vi "SetConf.vi"(8 "error in (no error)":errorcluster, 11 "BME68x in":refnum<class "BME680.lvclass">) -> (0 "error out":errorcluster, 3 "BME68x out":refnum<class "BME680.lvclass">)   [LabVIEW 2022 SP3, in "BME680.lvlib" / "BME680.lvclass"]
uses:
  BME680.lvclass
  BME680.lvclass/BME680.ctl
  Typedefs/Conf.ctl
panel:
  in  "Conf":T1
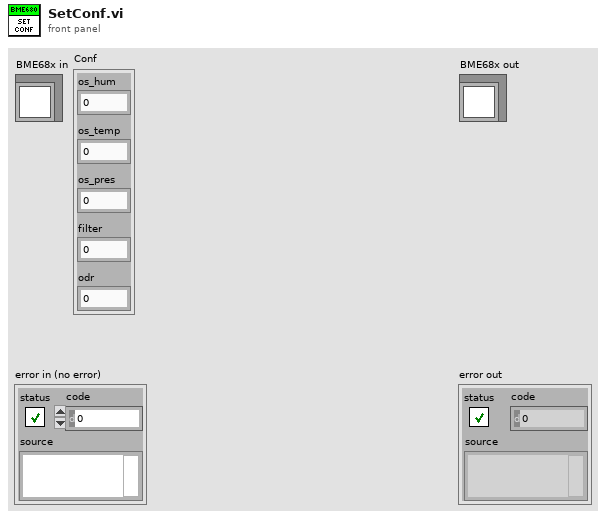
[diagram p1: front panel]
types:
  T1 = typedef "BME680.lvlib/BME680.lvclass/Conf.ctl" = cluster{"os_hum":u8, "os_temp":u8, "os_pres":u8, "filter":u8, "odr":u8}
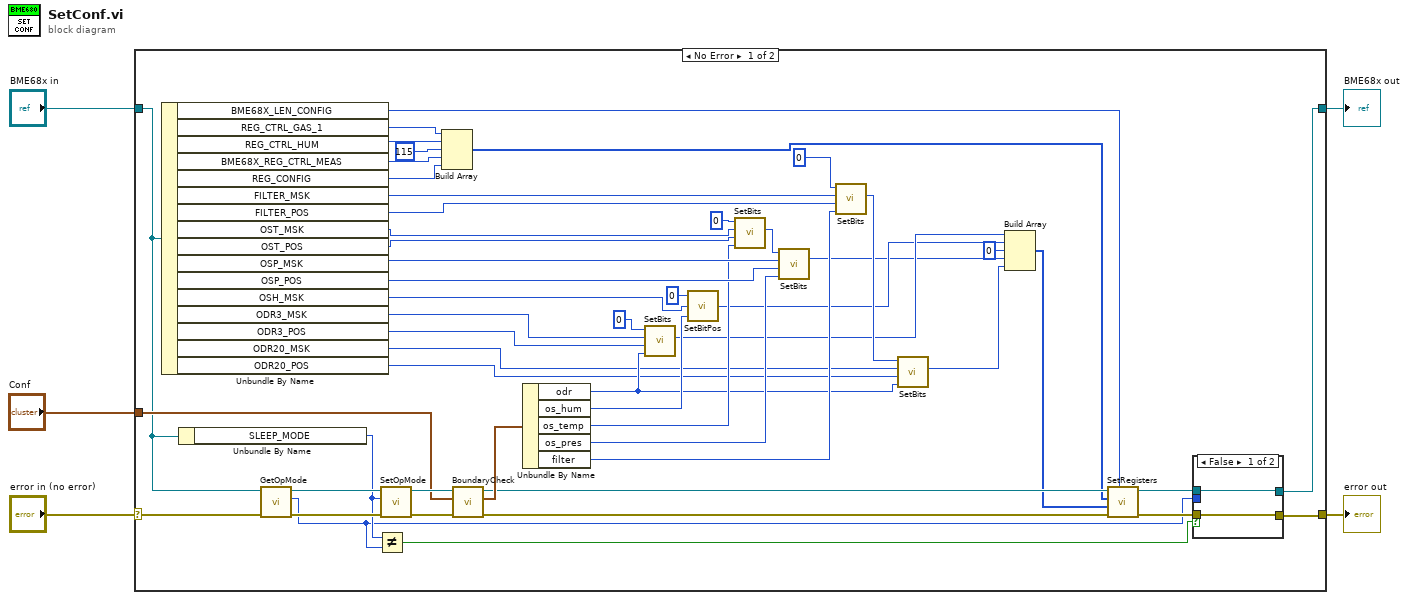
[diagram p0: block diagram]
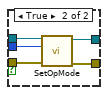
[diagram p2: hidden frame]
diagram:
  n1 = case shown="No Error" "error in (no error)" {
    selector: "error in (no error)" -> [w57 w66]
    tunnel: [w7 w66] -> w4
    tunnel: [w6 w65] -> w2
    tunnel: "BME68x in" -> [w51 w65]
    tunnel: "Conf" -> [w52 _]
    frame No Error {
      n2 = Unbundle By Name(w51) -> ("BME68X_LEN_CONFIG"=w15:u8, "REG_CTRL_GAS_1"=w50:u8, "REG_CTRL_HUM"=w49:u8, "BME68X_REG_CTRL_MEAS"=w48:u8, "REG_CONFIG"=w47:u8, "FILTER_MSK"=w42:u8, "FILTER_POS"=w41:u8, "OST_MSK"=w40:u8, "OST_POS"=w39:u8, "OSP_MSK"=w37:u8, "OSP_POS"=w36:u8, "OSH_MSK"=w34:u8, "ODR3_MSK"=w28:u8, "ODR3_POS"=w27:u8, "ODR20_MSK"=w26:u8, "ODR20_POS"=w25:u8)
      n3 = Unbundle By Name(w51) -> ("SLEEP_MODE"=w10:u8)
      n4 = call-dynamic "GetOpMode.vi"("error in (no error)"=w57, "BME680 in"=w51) -> ("error out"=w56:errorcluster, "Op Mode"=w9:u8, "BME680 out"=w55:refnum<class "BME680.lvclass">)  [unwired: 7 in]
      n5 = Not Equal?(x=w10, y=w9) -> (x != y?=w8:bool)
      n6 = call-dynamic "SetOpMode.vi"("error in (no error)"=w56, "Op Mode"=w10, "BME680 in"=w55) -> ("error out"=w54:errorcluster, "BME680 out"=w53:refnum<class "BME680.lvclass">)  [unwired: 7 in]
      n7 = Build Array(w50, w49, u8 115 ("element"), w48, w47) -> (w14:u8[])
      n8 = call "BoundaryCheck.vi"("error in (no error)"=w54, "Conf"=w52, "BME68x in"=w53) -> ("error out"=w17:errorcluster, "output cluster"=w46:T1, "BME68x out"=w16:refnum<class "BME680.lvclass">)  [unwired: 6 in]
      n9 = Unbundle By Name(w46) -> ("odr"=w29:u8, "os_hum"=w30:u8, "os_temp"=w31:u8, "os_pres"=w32:u8, "filter"=w33:u8)
      n10 = call "SetBits.vi"("Datain"=w29, "Pos"=w27, "Mask"=w28, "Reg data"=u8 0) -> ("Data"=w22:u16)  [unwired: 7 in]
      n11 = call "SetBitPos.vi"("Datain"=w30, "Mask"=w34, "Reg data"=u8 0) -> ("Data"=w20:u16)
      n12 = call "SetBits.vi"("Datain"=w31, "Pos"=w39, "Mask"=w40, "Reg data"=u8 0) -> ("Data"=w38:u16)  [unwired: 7 in]
      n13 = call "SetBits.vi"("Datain"=w32, "Pos"=w36, "Mask"=w37, "Reg data"=w38) -> ("Data"=w19:u16)  [unwired: 7 in]
      n14 = call "SetBits.vi"("Datain"=w33, "Pos"=w41, "Mask"=w42, "Reg data"=u8 0) -> ("Data"=w24:u16)  [unwired: 7 in]
      n15 = call "SetBits.vi"("Datain"=w29, "Pos"=w25, "Mask"=w26, "Reg data"=w24) -> ("Data"=w21:u16)  [unwired: 7 in]
      n16 = Build Array(w22, w20, u16 0 ("element"), w19, w21) -> (w13:u16[])
      n17 = call-dynamic "SetRegisters.vi"("Lenght"=w15, "error in (no error)"=w17, "Register Data"=w13, "Register Addres"=w14, "BME680 in"=w16) -> ("error out"=w12:errorcluster, "BME680 out"=w11:refnum<class "BME680.lvclass">)  [unwired: 5 in]
      n18 = case shown="False" w8 {
        tunnel: w9 -> [_ w64]
        tunnel: w12 -> [w59 w63]
        tunnel: w11 -> [w58 w62]
        tunnel: [w59 w61] -> w7
        tunnel: [w58 w60] -> w6
        frame False {
        }
        frame True {
          n19 = call-dynamic "SetOpMode.vi"("error in (no error)"=w63, "Op Mode"=w64, "BME680 in"=w62) -> ("error out"=w61:errorcluster, "BME680 out"=w60:refnum<class "BME680.lvclass">)  [unwired: 7 in]
        }
      }
    }
    frame Error {
    }
  }
  "error out" <- w4
  "BME68x out" <- w2
